vi "Set Test Properties.vi"(8 "error in":errorcluster, 11 "TDMS in":refnum<class "TDMS.lvclass">) -> (0 "error out":errorcluster, 3 "TDMS out":refnum<class "TDMS.lvclass">)   [LabVIEW 2019, in "TDMS.lvlib" / "TDMS.lvclass"]
uses:
  TDMS.lvclass
  C:/Users/Public/Documents/Development/builds/Tools/Report.lvlibp/Report.lvclass
  TDMS.lvclass/TDMS.ctl
  Accessors/Read TDMS Ref.vi
  Accessors/Write TDMS Ref.vi
  builds/Tools/Report.lvlibp/Accessors/Read Tester.vi
  builds/Tools/Report.lvlibp/Accessors/Read Witness.vi
  builds/Tools/Report.lvlibp/Accessors/Read Test Name.vi
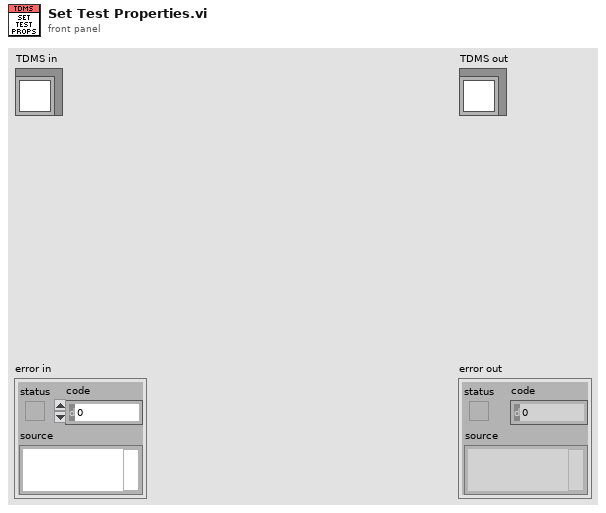
[diagram p1: front panel]
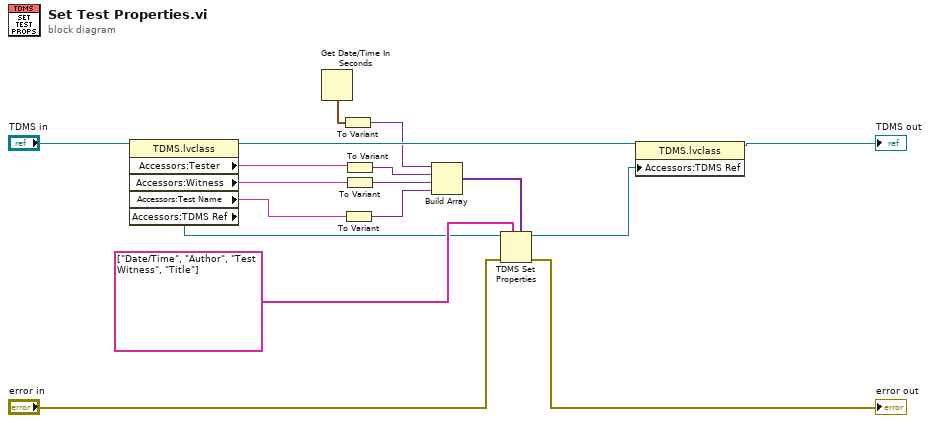
[diagram p0: block diagram]
diagram:
  n1 = property class="TDMS.lvclass"(reference="TDMS in") -> (reference out=w9:refnum<class "TDMS.lvclass">, "Accessors:Tester"=w16:string, "Accessors:Witness"=w15:string, "Accessors:Test Name"=w2:string, "Accessors:TDMS Ref"=w4:refnum<k34>)  [unwired: 1 in, 1 out]
  n2 = Get Date/Time In Seconds() -> (seconds since 1Jan1904=w5:timestamp)
  n3 = To Variant(anything=w5) -> (Variant=w3:variant)
  n4 = To Variant(anything=w2) -> (Variant=w1:variant)
  n5 = To Variant(anything=w16) -> (Variant=w14:variant)
  n6 = To Variant(anything=w15) -> (Variant=w13:variant)
  n7 = Build Array(w3, w14, w13, w1) -> (w12:variant[])
  n8 = TDMS Set Properties(5:w12, 7:string[] ["Date/Time", "Author", "Test Witness", "Title"], 8:"error in", 11:w4) -> (0:→"error out":errorcluster, 3:w7:refnum<k34>)  [unwired: 2 in, 2 out]
  n9 = property class="TDMS.lvclass"(reference=w9, "Accessors:TDMS Ref"=w7) -> (reference out=→"TDMS out":refnum<class "TDMS.lvclass">)  [unwired: 1 in, 1 out]
